vi "TCP URL and Resource Name.vi"() -> (2 "visa resource name":string, 3 "url":string)   [LabVIEW 2020, in "MeasurementServerTests.lvlib"]
uses:
  MeasurementServerTests.lvlib
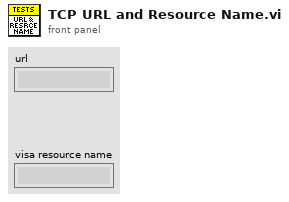
[diagram p1: front panel]
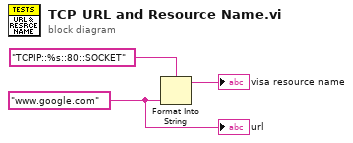
[diagram p0: block diagram]
diagram:
  w2 = "www.google.com"
  n1 = Format Into String(format string="TCPIP::%s::80::SOCKET" ("resource name"), w2) -> (resulting string=→"visa resource name":string)  [unwired: 2 in, 1 out]
  "url" <- w2
